vi "Pixel_Coords_To_Patch_Index.vi"(5 "Selected_Coreset_Element_Info":T1, 11 "Coords":cluster{"X":i32, "Y":i32}) -> (3 "Flat_Patch_Coords":i32)   [LabVIEW 2020]
uses:
  Controls/Selected_Coreset_Elements_and_Dim_Stride_Info.ctl
  Controls/Dims(2D)ctl.ctl
  <vilib>/Ngene/DeepLTK Anomaly Detection Addon/Toolkit/API/Controls/Feature_Coords(Idx,i,j).ctl
  <vilib>/Ngene/DeepLTK Anomaly Detection Addon/Toolkit/DeepLTK_Anomaly_Detection_Addon.lvlib
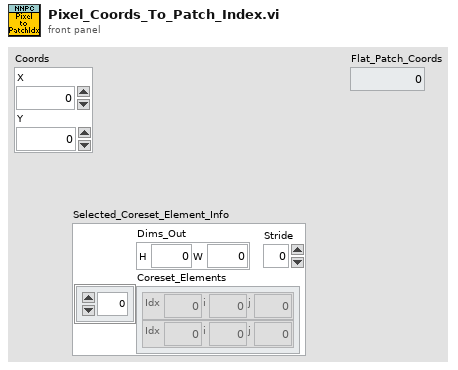
[diagram p1: front panel]
types:
  T1 = typedef "Selected_Coreset_Elements_and_Dim_Stride_Info.ctl" = cluster{"Dims_Out":T2, "Stride":i32, "Coreset_Elements":T3[]}
  T2 = typedef "Dims(2D)ctl.ctl" = cluster{"H":i32, "W":i32}
  T3 = typedef "DeepLTK_Anomaly_Detection_Addon.lvlib/Feature_Coords(Idx,i,j).ctl" = cluster{"Idx":i32, "i":i32, "j":i32}
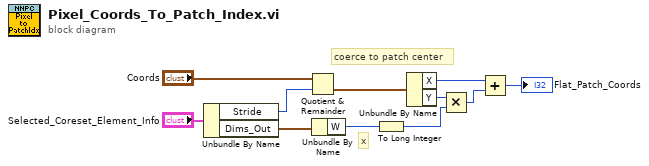
[diagram p0: block diagram]
diagram:
  # "x"
  # "coerce to patch center"
  n1 = Unbundle By Name("Selected_Coreset_Element_Info") -> ("Stride"=w1:i32, "Dims_Out"=w2:T2)
  n2 = Quotient & Remainder(x="Coords", y=w1) -> (floor(x/y)=w10:cluster{"X":i32, "Y":i32})  [unwired: 1 out]
  n3 = Unbundle By Name(w2) -> ("W"=w6:i32)
  n4 = To Long Integer(number=w6) -> (32bit integer=w4:i32)
  n5 = Unbundle By Name(w10) -> ("X"=w8:i32, "Y"=w7:i32)
  n6 = Multiply(x=w7, y=w4) -> (x*y=w9:i32)
  n7 = Add(x=w8, y=w9) -> (x+y=→"Flat_Patch_Coords":i32)
